vi "Input Monitor Reset.vi"(7 "Unit Address (1)":u8=1, 8 "error in (no error)":errorcluster, 10 "Selected Input Monitor (0: Input Monitor 1)":u8(ring) items=["Input monitor 1", "Input monitor 2"], 11 "VISA resource name":refnum<visa-resource-name>) -> (0 "error out":errorcluster, 3 "VISA resource name out":refnum<visa-resource-name>)   [LabVIEW 2014, in "Eurotherm 35xx Series.lvlib"]
doc: "This VI resets the Max and Min values and resets the time above threshold to zero."
uses:
  <instrlib>/Eurotherm 35xx Series/Eurotherm 35xx Series.lvlib
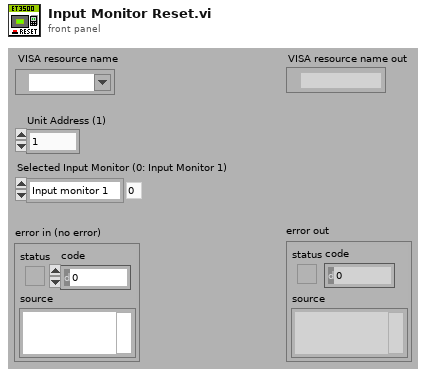
[diagram p1: front panel]
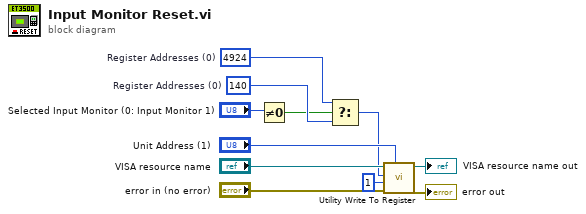
[diagram p0: block diagram]
diagram:
  w3 = 140  # Register Addresses (0)
  w4 = 4924  # Register Addresses (0)
  n1 = Not Equal To 0?(x="Selected Input Monitor (0: Input Monitor 1)") -> (x != 0?=w2:bool)
  n2 = Select(t=w4, s=w2, f=w3) -> (s? t:f=w1:i32)
  n3 = call <instrlib>:"Utility Write To Register.vi"("Unit Address (1)"="Unit Address (1)", "error in (no error)"="error in (no error)", "Data (0)"=i16 1, "Register Address (0)"=w1, "VISA resource name"="VISA resource name") -> ("error out"=→"error out":errorcluster, "VISA resource name out"=→"VISA resource name out":refnum<visa-resource-name>)  [unwired: 5 in]
